vi "SimpleAlarm.vi"(7 "ResetAlarm":bool, 9 "Enable":bool, 11 "AlarmCondition":bool) -> (3 "Alarm":bool)   [LabVIEW 2019]
doc: "Simple lock for alarm.\n<b>AlarmCondition</b> can cause an <b>Alarm</b> while <b>Enable</b> is True"
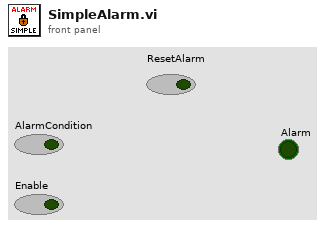
[diagram p1: front panel]
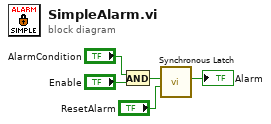
[diagram p0: block diagram]
diagram:
  n1 = And(x="AlarmCondition", y="Enable") -> (x .and. y?=w4:bool)
  n2 = call "Synchronous Latch.vi"("reset"="ResetAlarm", "set"=w4) -> ("out"=→"Alarm":bool)  [unwired: 9 in]
